vi "PQfetchColumnNames.vi"(6 "error in":errorcluster, 8 "res":u32, 9 "conn":u32) -> (0 "error out":errorcluster, 1 "ColumnNames":string[](array[string]), 2 "res_out":u32, 3 "conn_out":u32)   [LabVIEW 2019, in "libpqutility.lvlib"]
doc: "Fetch Column Names for Result.\nSee PostgreSQL c-lib doku for further information."
uses:
  libpqutility.lvlib
  libpqlv/libpqlv.lvlib
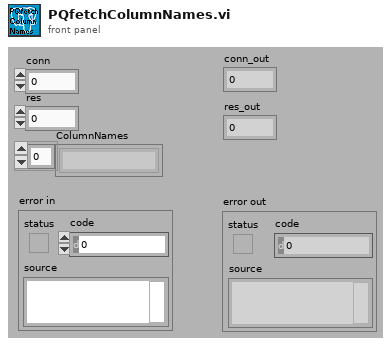
[diagram p1: front panel]
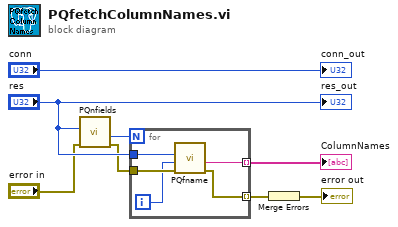
[diagram p0: block diagram]
diagram:
  n1 = call "PQnfields.vi"("error in (no error)"="error in", "res"="res") -> ("error out"=w3:errorcluster, "PQnFields"=w5:i32)  [unwired: 7 in, 1 out]
  n2 = for {
    N: w5 -> [_]
    tunnel: [w12] -> w8 mode=indexing
    tunnel: "res" -> [w13]
    tunnel: w3 -> [w11]
    tunnel: [w10] -> w2 mode=indexing
    i -> [w9]
    n3 = call "PQfname.vi"("error in (no error)"=w11, "cloumn_num"=w9, "res"=w13) -> ("error out"=w10:errorcluster, "ColumnName"=w12:string)  [unwired: 4 in, 1 out]
  }
  "ColumnNames" <- w8
  n4 = Merge Errors(w2) -> (→"error out":errorcluster)
  "res_out" <- "res"
  "conn_out" <- "conn"
